vi "SubVI PID.vi"(8 "error in (no error)":errorcluster, 11 "Image Src":T1) -> (0 "Number of Matches (Color Location 2)":i32, 1 "Number of Matches (Color Location 1)":i32, 2 "Classes (Color Classification 1)":string[](array[string]), 3 "String (OCR/OCV 1)":string)   [LabVIEW 2019, in "Analisis.lvlib"]
uses:
  Analisis.lvlib
  <vilib>/vision/Image Controls.llb/IMAQ Image.ctl
  <vilib>/vision/Classification.llb/IMAQ Classifier Read Options.ctl
  <vilib>/vision/NI_Vision_Development_Module.lvlib
panel:
  out "error out":errorcluster
  out "Image Out":T1(plugin-control)
  out "Matches (calibrated) (Color Location 2)":T2(array[cluster]) {"Bounding Box"."y" format="%.2f"; "Bounding Box"."x" format="%.2f"; "Position"."y" format="%.2f"; "Position"."x" format="%.2f"; "Score" format="%.2f"; "Scale" format="%.2f"; "Angle" format="%.2f"}
  out "Matches (Color Location 2)":T2(array[cluster]) {"Bounding Box"."y" format="%.2f"; "Bounding Box"."x" format="%.2f"; "Position"."y" format="%.2f"; "Position"."x" format="%.2f"; "Score" format="%.2f"; "Scale" format="%.2f"; "Angle" format="%.2f"}
  out "Matches (calibrated) (Color Location 1)":T2(array[cluster]) {"Bounding Box"."y" format="%.2f"; "Bounding Box"."x" format="%.2f"; "Position"."y" format="%.2f"; "Position"."x" format="%.2f"; "Score" format="%.2f"; "Scale" format="%.2f"; "Angle" format="%.2f"}
  out "Matches (Color Location 1)":T2(array[cluster]) {"Bounding Box"."y" format="%.2f"; "Bounding Box"."x" format="%.2f"; "Position"."y" format="%.2f"; "Position"."x" format="%.2f"; "Score" format="%.2f"; "Scale" format="%.2f"; "Angle" format="%.2f"}
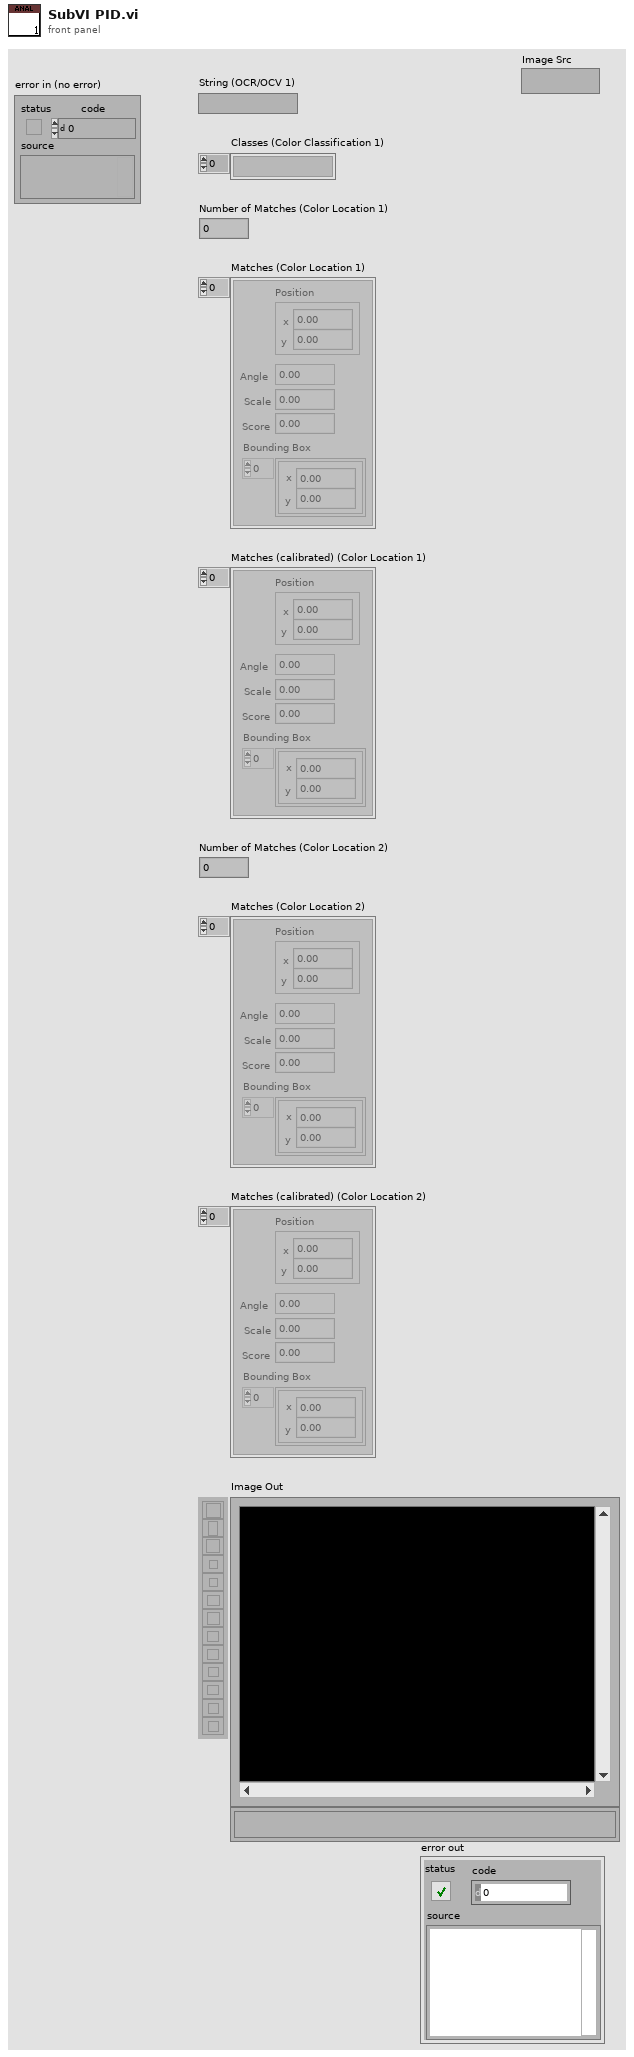
[diagram p1: front panel]
types:
  T1 = typedef "IMAQ Image.ctl" = refnum<image>
  T2 = cluster{"Position":cluster{"x":sgl, "y":sgl}, "Angle":sgl, "Scale":sgl, "Score":sgl, "Bounding Box":cluster{"x":sgl, "y":sgl}[]}[]
  T3 = typedef "Image Type" = u32
  T4 = cluster{"Global Rectangle":i32[], "Contours":cluster{"ID":enum32{"External", "Internal"}, "Type":u32, "Coordinates":i32[]}[]}
  T5 = cluster{"Threshold Data":cluster{"Method":enum16{"Fixed Range", "Uniform", "Linear", "Non Linear", "Local", "Color"}, "Looking for":u32, "Color Mode":u32, "Kernel Size":cluster{"Width":i32, "Height":i32}, "Ranges":cluster{"Min":i32, "Max":i32}[]}, "Reject Border":bool, "Number Of Erosions":i32, "Size & Spacing":cluster{"Segment Algorithm":u16, "Min Bounding Rect Width":i32, "Max Bounding Rect Width":i32, "Min Bounding Rect Height":i32, "Max Bounding Rect Height":i32, "Min Character Size":i32, "Max Character Size":i32, "Min Char Spacing":i32, "Max Horiz Element Spacing":i32, "Max Vert Element Spacing":i32, "Max Space Distance":i32}, "Read Options":cluster{"Read Strategy":i32, "Read Resolution":i32, "Scale Dependant":bool, "Aspect Ratio":i32, "Acceptance Level":i32, "Substitution Character":string, "MultiLine":bool}, "Valid Characters":cluster{"Pre-defined characters":i32, "User-defined characters":string}[], "Use Text Pattern":bool, "Orientation":u32, "# Lines Expected":u32, "Number of Blocks":i32}
  T6 = typedef "IMAQ OCR Session.ctl" = refnum<k1>
  T7 = typedef "IMAQ Classifier Read Options.ctl" = i32
  T8 = typedef "IMAQ Classifier Session.ctl" = refnum<k1>
  T9 = typedef "ROI Descriptor" = cluster{"Global Rectangle":i32[], "Contours":cluster{"ID":enum32{"External", "Internal"}, "Type":u32, "Coordinates":i32[]}[]}
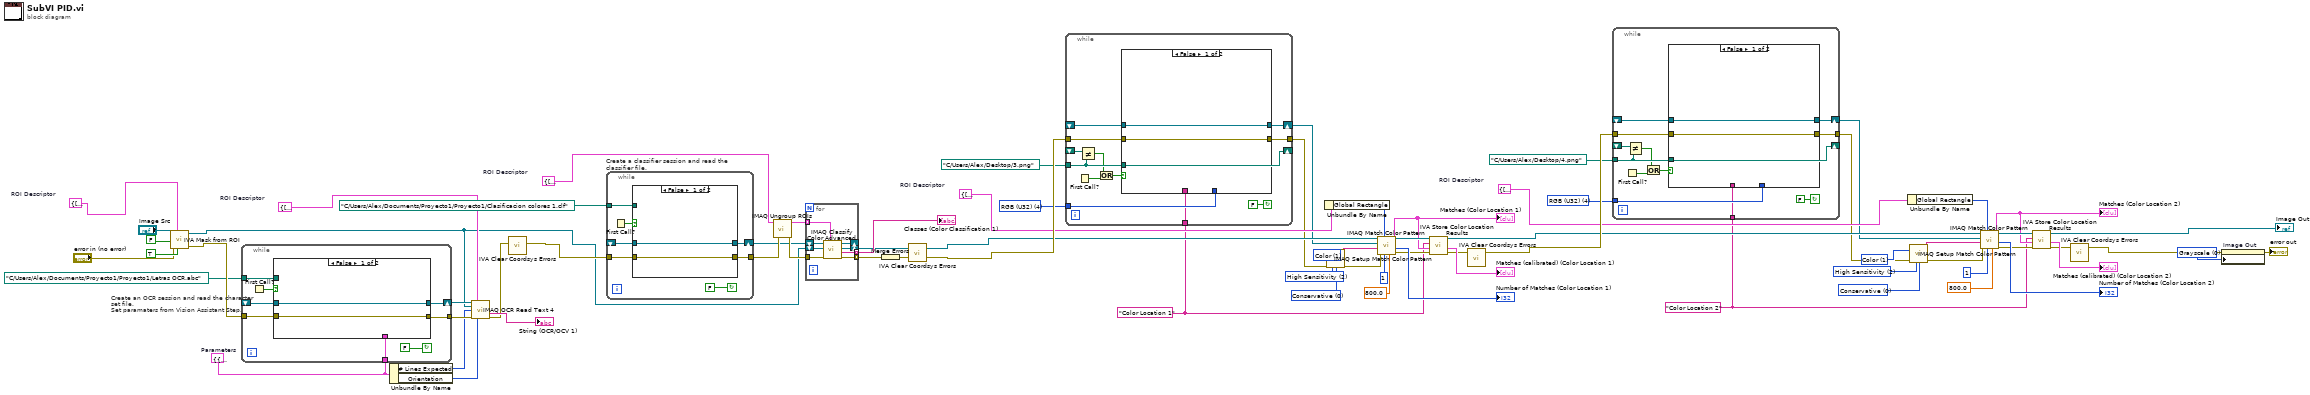
[diagram p0: block diagram]
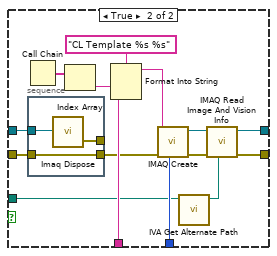
[diagram p2: hidden frame]
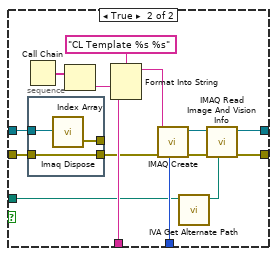
[diagram p3: hidden frame]
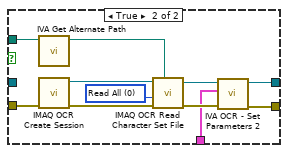
[diagram p4: hidden frame]
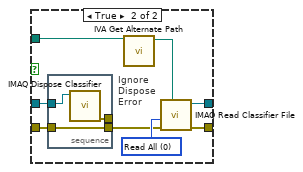
[diagram p5: hidden frame]
diagram:
  w4 = u32 0 items=["Grayscale", "Binary", "Gradient", "Rainbow", "Temperature", "User Defined", "Binary 16 Bit", "Gradient 16 Bit", "Rainbow 16 Bit", "Temperature 16 Bit", "User Defined 16 Bit"] ("Palette Type")
  w13 = "Color Location 2" ("Step Name")
  w19 = T3 4 items=["Grayscale (U8)", "Grayscale (I16)", "Grayscale (SGL)", "Complex (CSG)", "RGB (U32)", "HSL (U32)", "RGB (U64)"] ("Image Type")
  w21 = u32 0 items=["Conservative", "Balance", "Aggressive", "Very Aggressive"] ("Search Strategy")
  w22 = u32 2 items=["Low Sensitivity", "Medium Sensitivity", "High Sensitivity"] ("Color Sensitivity")
  w23 = u32 1 items=["Color and Shape", "Color", "Shape"] ("Match Feature Mode")
  w18 = T4 {"Global Rectangle"=[160, 1248, 1380, 1764], "Contours"=[{"ID"=enum."External", "Type"=12, "Coordinates"=[160, 1248, 1380, 1764, 0]}]}  # ROI Descriptor
  w34 = "Color Location 1" ("Step Name")
  w40 = T3 4 items=["Grayscale (U8)", "Grayscale (I16)", "Grayscale (SGL)", "Complex (CSG)", "RGB (U32)", "HSL (U32)", "RGB (U64)"] ("Image Type")
  w42 = u32 0 items=["Conservative", "Balance", "Aggressive", "Very Aggressive"] ("Search Strategy")
  w43 = u32 2 items=["Low Sensitivity", "Medium Sensitivity", "High Sensitivity"] ("Color Sensitivity")
  w44 = u32 1 items=["Color and Shape", "Color", "Shape"] ("Match Feature Mode")
  w39 = T4 {"Global Rectangle"=[156, 1256, 1312, 1764], "Contours"=[{"ID"=enum."External", "Type"=12, "Coordinates"=[156, 1256, 1312, 1764, 0]}]}  # ROI Descriptor
  w56 = T4 {"Global Rectangle"=[252, 252, 1224, 504], "Contours"=[{"ID"=enum."External", "Type"=3, "Coordinates"=[252, 252, 1224, 504]}]}  # ROI Descriptor
  w65 = T5 {"Threshold Data"={"Method"=enum."Color", "Looking for"=1, "Color Mode"=0, "Kernel Size"={"Width"=32, "Height"=32}, "Ranges"=[{"Min"=0, "Max"=53}, {"Min"=0, "Max"=90}, {"Min"=0, "Max"=128}]}, "Reject Border"=TRUE, "Number Of Erosions"=0, "Size & Spacing"={"Segment Algorithm"=0, "Min Bounding Rect Width"=1, "Max Bounding Rect Width"=65536, "Min Bounding Rect Height"=1, "Max Bounding Rect Height"=65536, "Min Character Size"=500, "Max Character Size"=65536, "Min Char Spacing"=1, "Max Horiz Element Spacing"=1, "Max Vert Element Spacing"=0, "Max Space Distance"=65536}, "Read Options"={"Read Strategy"=1, "Read Resolution"=2, "Scale Dependant"=FALSE, "Aspect Ratio"=400, "Acceptance Level"=700, "Substitution Character"="?", "MultiLine"=TRUE}, "Valid Characters"=[], "Use Text Pattern"=FALSE, "Orientation"=0, "# Lines Expected"=0, "Number of Blocks"=4}  # Parameters
  w66 = T4 {"Global Rectangle"=[202, 773, 1267, 1097], "Contours"=[{"ID"=enum."External", "Type"=3, "Coordinates"=[202, 773, 1267, 1097]}]}  # ROI Descriptor
  w72 = T4 {"Global Rectangle"=[1175, 235, 2635, 2095], "Contours"=[{"ID"=enum."External", "Type"=3, "Coordinates"=[1175, 235, 2635, 2095]}]}  # ROI Descriptor
  n1 = call <vilib>:"IVA Mask from ROI.vi"("Shrink"=TRUE, "ROI Descriptor"=w72, "error in (no error)"="error in (no error)", "Out / In"=FALSE, "Image Src"="Image Src") -> ("error out"=w69:errorcluster, "Image Out"=w49:T1)  [unwired: 5 out]
  n2 = while "Create an OCR session and read the character set file.\nSet paramaters from Vision Assistant Step." {
    shift-right: [w77] -> w63
    shift-left: _ -> [w76]
    tunnel: w69 -> [w79]
    tunnel: w65 -> [w75]
    tunnel: path "C:/Users/Alex/Documents/Proyecto1/Proyecto1/Letras OCR.abc" ("File Path") -> [w74]
    tunnel: [w73] -> w64
    stop <- FALSE continue-if-true
    n3 = First Call?() -> (First Call?: T/F=w78:bool)
    n4 = case shown="False" w78 {
      tunnel: w74 -> [_ w86]
      tunnel: w79 -> [w81 w90]
      tunnel: [w82 w88] -> w77
      tunnel: [w81 w87] -> w73
      tunnel: w75 -> [_ w83]
      tunnel: w76 -> [w82 _]
      frame False {
      }
      frame True {
        w91 = 0 items=["Read All", "Read Character Set Only", "Read Properties Only"] ("Read Options")
        n5 = call <vilib>:"IVA Get Alternate Path.vi"("Path In"=w86) -> ("Path Out"=w85:path)  [unwired: 10 out]
        n6 = call "IMAQ OCR Create Session"("error in (no error)"=w90) -> ("error out"=w92:errorcluster, "IMAQ OCR Session"=w93:T6)  [unwired: 9 out]
        n7 = call "IMAQ OCR Read Character Set File"("File Path"=w85, "error in (no error)"=w92, "Read Options"=w91, "IMAQ OCR Session"=w93) -> ("error out"=w89:errorcluster, "IMAQ OCR Session (dup)"=w84:T6)  [unwired: 1 in, 5 out]
        n8 = call <vilib>:"IVA OCR - Set Parameters 2.vi"("error in (no error)"=w89, "Parameters"=w83, "IMAQ OCR Session"=w84) -> ("error out"=w87:errorcluster, "IMAQ OCR Session Out"=w88:T6)  [unwired: 7 in]
      }
    }
  }
  n9 = Unbundle By Name(w65) -> ("# Lines Expected"=w61:u32, "Orientation"=w62:u32)
  n10 = call "IMAQ OCR Read Text 4"("IMAQ OCR Session"=w63, "ROI Descriptor"=w66, "Image"=w49, "Number of Lines Requested"=w61, "error in (no error)"=w64, "Orientation"=w62) -> ("Read String"=→"String (OCR/OCV 1)":string, "error out"=w60:errorcluster)  [unwired: 8 out]
  n11 = call <vilib>:"IVA Clear Coordsys Errors.vi"("error in (no error)"=w60) -> ("error out"=w59:errorcluster)  [unwired: 10 in]
  n12 = while "Create a classifier session and read the classifier file." {
    shift-right: [w100] -> w48
    shift-left: _ -> [w99]
    tunnel: w59 -> [w97]
    tunnel: [w96] -> w55
    tunnel: path "C:/Users/Alex/Documents/Proyecto1/Proyecto1/Clasificacion colores 1.clf" ("File Path") -> [w95]
    stop <- FALSE continue-if-true
    n13 = First Call?() -> (First Call?: T/F=w94:bool)
    n14 = case shown="False" w94 {
      tunnel: [w102 w109] -> w100
      tunnel: w99 -> [w102 w107]
      tunnel: w97 -> [w101 w106]
      tunnel: [w101 w108] -> w96
      tunnel: w95 -> [_ w104]
      frame False {
      }
      frame True {
        w110 = T7 0 items=["Read All", "Add Samples, Do Not Change Options", "Read Options, Do Not Add Samples"] ("Read Options")
        # "Ignore Dispose Error"
        n15 = stacked-sequence {
          tunnel: w107 -> [w113]
          tunnel: w106 -> [w112]
          tunnel: [w112] -> w105
          tunnel: [w111] -> _
          frame #0 {
            n16 = call "IMAQ Dispose Classifier"("Classifier Session"=w113) -> ("error out"=w111:errorcluster)  [unwired: 1 in, 9 out]
          }
        }
        n17 = call <vilib>:"IVA Get Alternate Path.vi"("Path In"=w104) -> ("Path Out"=w103:path)  [unwired: 10 out]
        n18 = call "IMAQ Read Classifier File"("File Path"=w103, "error in (no error)"=w105, "Read Options"=w110) -> ("error out"=w108:errorcluster, "Classifier Session"=w109:T8)  [unwired: 1 in, 6 out]
      }
    }
  }
  n19 = call "IMAQ Ungroup ROIs"("error in (no error)"=w55, "ROI Descriptor"=w56) -> ("error out"=w54:errorcluster, "ROI Descriptors out"=w53:T9[])  [unwired: 2 out]
  n20 = for {
    tunnel: [w121] -> w57 mode=indexing
    tunnel: [w120] -> w52 mode=indexing
    tunnel: w54 -> [w118]
    tunnel: w53 -> [w117] mode=indexing
    shift-right: [w115] -> w36
    shift-left: w49 -> [w116]
    shift-right: [w114] -> _
    shift-left: w48 -> [w119]
    n21 = call "IMAQ Classify Color Advanced"("ROI Descriptor"=w117, "error in (no error)"=w118, "Image"=w116, "Classifier Session"=w119) -> ("error out"=w120:errorcluster, "Class"=w121:string, "Image (dup)"=w115:T1, "Classifier Session (dup)"=w114:T8)  [unwired: 4 out]
  }
  "Classes (Color Classification 1)" <- w57
  n22 = Merge Errors(w52) -> (w51:errorcluster)
  n23 = call <vilib>:"IVA Clear Coordsys Errors.vi"("error in (no error)"=w51) -> ("error out"=w50:errorcluster)  [unwired: 10 in]
  n24 = while {
    shift-right: [w133] -> w30
    shift-left: _ -> [w132]
    tunnel: [w130] -> w29
    tunnel: w50 -> [w129]
    tunnel: path "C:/Users/Alex/Desktop/3.png" ("File Path") -> [w125]
    tunnel: w40 -> [w128]
    tunnel: w34 -> [w127]
    shift-right: [w125] -> _
    shift-left: _ -> [w126]
    stop <- FALSE continue-if-true
    n25 = First Call?() -> (First Call?: T/F=w124:bool)
    n26 = Not Equal?(x=w126, y=w125) -> (x != y?=w123:bool)
    n27 = Or(x=w123, y=w124) -> (x .or. y?=w122:bool)
    n28 = case shown="False" w122 {
      tunnel: [w135 w148] -> w133
      tunnel: w132 -> [w135 w140]
      tunnel: [w134 w145] -> w130
      tunnel: w129 -> [w134 w139]
      tunnel: w128 -> [_ w144]
      tunnel: w127 -> [_ w141]
      tunnel: w125 -> [_ w137]
      frame False {
      }
      frame True {
        n29 = Call Chain() -> (call chain=w143:string[])
        n30 = stacked-sequence {
          tunnel: w140 -> [w153]
          tunnel: w139 -> [w152]
          tunnel: [w152] -> w138
          tunnel: [w151] -> _
          frame #0 {
            n31 = call "Imaq Dispose"("Image"=w153) -> ("error out"=w151:errorcluster)  [unwired: 2 in, 3 out]
          }
        }
        n32 = Index Array(array=w143) -> (element=w142:string)  [unwired: 1 in]
        n33 = Format Into String(format string="CL Template %s %s" ("Image Name"), w142, w141) -> (resulting string=w150:string)  [unwired: 2 in, 1 out]
        n34 = call "IMAQ Create"("Image Name"=w150, "Image Type"=w144, "error in (no error)"=w138) -> ("New Image"=w147:T1, "error out"=w146:errorcluster)  [unwired: 1 in, 1 out]
        n35 = call <vilib>:"IVA Get Alternate Path.vi"("Path In"=w137) -> ("Path Out"=w136:path)  [unwired: 10 out]
        n36 = call "IMAQ Read Image And Vision Info"("File Path"=w136, "error in (no error)"=w146, "Image"=w147) -> ("error out"=w145:errorcluster, "Image Out"=w148:T1)  [unwired: 1 in, 6 out]
      }
    }
  }
  n37 = Unbundle By Name(w39) -> ("Global Rectangle"=w31:i32[])
  n38 = call "IMAQ Setup Match Color Pattern"("Match Feature Mode"=w44, "error in (no error)"=w29, "Color Sensitivity"=w43, "Search Strategy"=w42) -> ("Match Color Pattern Setup Data"=w33:string, "error out"=w32:errorcluster)  [unwired: 5 in, 5 out]
  n39 = call "IMAQ Match Color Pattern"("Minimum Match Score"=sgl 800.0, "Number of Matches Requested"=1, "Optional Rectangle"=w31, "error in (no error)"=w32, "Match Color Pattern Setup Data"=w33, "Template Image"=w30, "Image"=w36) -> ("error out"=w37:errorcluster, "Number of Matches"=→"Number of Matches (Color Location 1)":i32, "Matches"=w35:T2)  [unwired: 2 out]
  "Matches (Color Location 1)" <- w35
  n40 = call <vilib>:"IVA Store Color Location Results.vi"("error in (no error)"=w37, "Matches"=w35, "Step Name"=w34, "Image in"=w36) -> ("error out"=w28:errorcluster, "Calibrated Matches"=→"Matches (calibrated) (Color Location 1)":T2, "Image dup"=w15:T1)  [unwired: 5 out]
  n41 = call <vilib>:"IVA Clear Coordsys Errors.vi"("error in (no error)"=w28) -> ("error out"=w27:errorcluster)  [unwired: 10 in]
  n42 = while {
    shift-right: [w165] -> w9
    shift-left: _ -> [w164]
    tunnel: [w162] -> w8
    tunnel: w27 -> [w161]
    tunnel: path "C:/Users/Alex/Desktop/4.png" ("File Path") -> [w157]
    tunnel: w19 -> [w160]
    tunnel: w13 -> [w159]
    shift-right: [w157] -> _
    shift-left: _ -> [w158]
    stop <- FALSE continue-if-true
    n43 = First Call?() -> (First Call?: T/F=w156:bool)
    n44 = Not Equal?(x=w158, y=w157) -> (x != y?=w155:bool)
    n45 = Or(x=w155, y=w156) -> (x .or. y?=w154:bool)
    n46 = case shown="False" w154 {
      tunnel: [w167 w180] -> w165
      tunnel: w164 -> [w167 w172]
      tunnel: [w166 w177] -> w162
      tunnel: w161 -> [w166 w171]
      tunnel: w160 -> [_ w176]
      tunnel: w159 -> [_ w173]
      tunnel: w157 -> [_ w169]
      frame False {
      }
      frame True {
        n47 = Call Chain() -> (call chain=w175:string[])
        n48 = stacked-sequence {
          tunnel: w172 -> [w185]
          tunnel: w171 -> [w184]
          tunnel: [w184] -> w170
          tunnel: [w183] -> _
          frame #0 {
            n49 = call "Imaq Dispose"("Image"=w185) -> ("error out"=w183:errorcluster)  [unwired: 2 in, 3 out]
          }
        }
        n50 = Index Array(array=w175) -> (element=w174:string)  [unwired: 1 in]
        n51 = Format Into String(format string="CL Template %s %s" ("Image Name"), w174, w173) -> (resulting string=w182:string)  [unwired: 2 in, 1 out]
        n52 = call "IMAQ Create"("Image Name"=w182, "Image Type"=w176, "error in (no error)"=w170) -> ("New Image"=w179:T1, "error out"=w178:errorcluster)  [unwired: 1 in, 1 out]
        n53 = call <vilib>:"IVA Get Alternate Path.vi"("Path In"=w169) -> ("Path Out"=w168:path)  [unwired: 10 out]
        n54 = call "IMAQ Read Image And Vision Info"("File Path"=w168, "error in (no error)"=w178, "Image"=w179) -> ("error out"=w177:errorcluster, "Image Out"=w180:T1)  [unwired: 1 in, 6 out]
      }
    }
  }
  n55 = Unbundle By Name(w18) -> ("Global Rectangle"=w10:i32[])
  n56 = call "IMAQ Setup Match Color Pattern"("Match Feature Mode"=w23, "error in (no error)"=w8, "Color Sensitivity"=w22, "Search Strategy"=w21) -> ("Match Color Pattern Setup Data"=w12:string, "error out"=w11:errorcluster)  [unwired: 5 in, 5 out]
  n57 = call "IMAQ Match Color Pattern"("Minimum Match Score"=sgl 800.0, "Number of Matches Requested"=1, "Optional Rectangle"=w10, "error in (no error)"=w11, "Match Color Pattern Setup Data"=w12, "Template Image"=w9, "Image"=w15) -> ("error out"=w16:errorcluster, "Number of Matches"=→"Number of Matches (Color Location 2)":i32, "Matches"=w14:T2)  [unwired: 2 out]
  "Matches (Color Location 2)" <- w14
  n58 = call <vilib>:"IVA Store Color Location Results.vi"("error in (no error)"=w16, "Matches"=w14, "Step Name"=w13, "Image in"=w15) -> ("error out"=w7:errorcluster, "Calibrated Matches"=→"Matches (calibrated) (Color Location 2)":T2, "Image dup"=→"Image Out":T1)  [unwired: 5 out]
  n59 = call <vilib>:"IVA Clear Coordsys Errors.vi"("error in (no error)"=w7) -> ("error out"=w6:errorcluster)  [unwired: 10 in]
  n60 = property on="Image Out" class="ImageControl"(error in=w6, "Palette:Palette Type"=w4) -> (error out=→"error out":errorcluster)  [unwired: 1 in, 1 out]
